vi "test_Add Array Format.vi"(8 "error in (no error)":errorcluster, 11 "TestCase in":refnum<class "Instrument Addon Scripting API Channels Unit Tests.lvclass">) -> (0 "error out":errorcluster, 3 "TestCase out":refnum<class "Instrument Addon Scripting API Channels Unit Tests.lvclass">)   [LabVIEW 2018, in "Instrument Addon Scripting API Channels Unit Tests.lvclass"]
uses:
  Instrument Addon Scripting API Channels Unit Tests.lvclass
  APIs/Scripting API/TypeDefs/Array Format Settings.ctl
  APIs/Scripting API/TypeDefs/Array Element.ctl
  Addon/Addon Shared/Types/Protocol Data Type.ctl
  Addon/Addon Shared/Types/Data Channel Type.ctl
  Instrument Addon Scripting API Channels Unit Tests.lvclass/Instrument Addon Scripting API Channels Unit Tests.ctl
  Addon/Addon Shared/SubVIs/Constants.vi
  <vilib>/NI/NI VeriStand Advanced SysDef API/_SubVIs/SysDef.Search.GUID.vi
  <vilib>/NI/NI VeriStand Advanced SysDef API/_SubVIs/SysDef.Search.GUIDs.vi
  APIs/Scripting API/Channels/Create Data Channel - Array - Format.vi
  <vilib>/NI Veristand/Custom Device API/Get Item Property (U16).vi
  <vilib>/NI Veristand/Custom Device API/Get Item Property (String).vi
  <vilib>/addons/_JKI Toolkits/VI Tester/TestCase.llb/TestCase.lvclass
  Instrument Addon Scripting API Test Assets/Instrument Addon Scripting API Test Assets.lvclass
  <vilib>/NI/NI VeriStand Advanced SysDef API/SysDef API/Advanced System Definition.lvlib
  Addon/Addon Shared/Instrument Addon Shared.lvlib
  APIs/Scripting API/Instrument Addon Scripting API.lvlib
  <vilib>/NI Veristand/Custom Device API/Custom Device API.lvlib
  C:/Program Files (x86)/National Instruments/LabVIEW 2018/vi.lib/addons/_JKI Toolkits/VI Tester/TestCase.llb/TestCase.lvclass
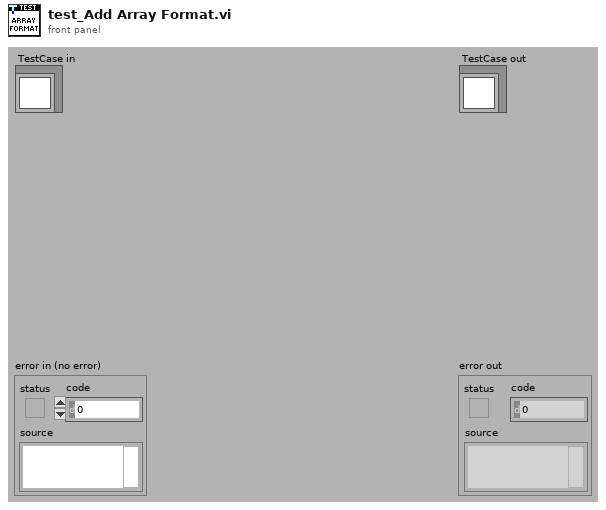
[diagram p1: front panel]
types:
  T1 = typedef "Instrument Addon Scripting API.lvlib/Array Format Settings.ctl" = cluster{"Elements":T2[], "Format String":string, "Delimiter":string}
  T2 = typedef "Instrument Addon Scripting API.lvlib/Array Element.ctl" = cluster{"Name":string, "Default Value":dbl, "Units":string}
  T3 = typedef "Instrument Addon Shared.lvlib/Data Channel Type.ctl" = enum16{"Format", "Comparison", "Type Cast", "Enumerated List"}
  T4 = typedef "Instrument Addon Shared.lvlib/Protocol Data Type.ctl" = enum16{"Single Channel", "Array"}
  T5 = typedef "Custom Device API.lvlib/Custom Device Item Ref.ctl" = u64
  T6 = typedef "Advanced System Definition.lvlib/TreeItem.Info.ctl" = cluster{"Name":string, "Description":string, "GUID":string, "Is Channel":bool, "Channel":T7, "Is Waveform":bool, "Waveform":T9}
  T7 = typedef "Custom Device API.lvlib/Custom Device Channel.ctl" = cluster{"Type":T8, "Units":string, "Default Value":dbl, "Faultable":bool, "Scalable":bool}
  T8 = typedef "Custom Device API.lvlib/Custom Device Channel Type.ctl" = enum16{"Input", "Output"}
  T9 = typedef "Custom Device API.lvlib/Custom Device Waveform.ctl" = cluster{"Data Type":T10, "Units":string}
  T10 = typedef "Custom Device API.lvlib/Custom Device Waveform DataType.ctl" = enum16{"Double", "Complex Double"}
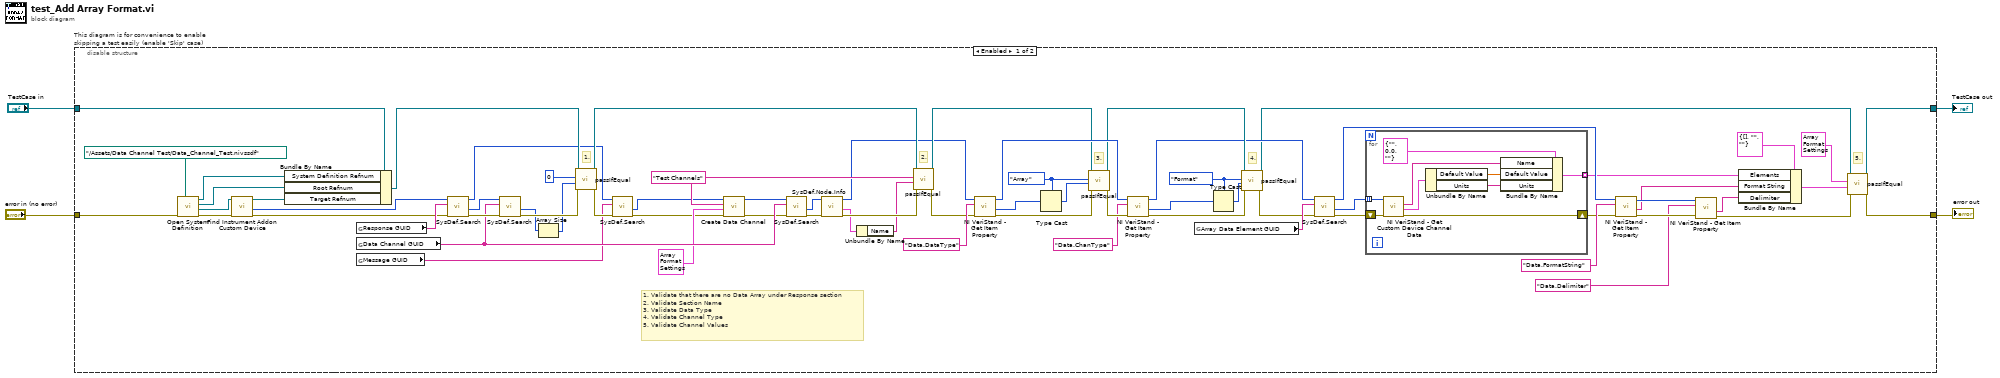
[diagram p0: block diagram]
diagram:
  n1 = disable-structure "This diagram is for convenience to enable skipping a test easily (enable 'Skip' case)" shown="Enabled" {
    disable-tunnel: "TestCase in" -> [w36 w88]
    disable-tunnel: [w49 w86] -> w1
    disable-tunnel: [w50 w87] -> w3
    disable-tunnel: "error in (no error)" -> [w72 w85]
    frame Enabled {
      w14 = Data_Channel_Type."Format" ("Channel Type")
      w19 = Protocol_Data_Type."Array" ("Data Type")
      w61 = "Test Channels" ("Name")
      # "1. Validate that there are no Data Array under Response section\n2. Validate Section Name\n3. Validate Data Type\n4. Validate Channel Type\n5. Validate Channel Values"
      # "4."
      # "3."
      # "5."
      # "2."
      # "1."
      n2 = call "Open System Definition.vi"("error in (no error)"=w72, "System Definition File"=path "../Assets/Data Channel Test/Data_Channel_Test.nivssdf") -> ("error out"=w75:errorcluster, "Target Refnum"=w74:refnum<k24>, "Root Refnum"=w34:refnum<k24>, "System Definition Refnum"=w35:refnum<k24>)  [unwired: 6 in]
      n3 = call "Find Instrument Addon Custom Device.vi"("error in"=w75, "target in"=w74) -> ("error out"=w32:errorcluster, "NodeID"=w71:u64, "target out"=w33:refnum<k24>)  [unwired: 7 in]
      n4 = Bundle By Name(cluster=w36, "System Definition Refnum"=w35, "Root Refnum"=w34, "Target Refnum"=w33) -> (w31:refnum<class "Instrument Addon Scripting API Channels Unit Tests.lvclass">)
      n5 = global read "Constants.vi" "Response GUID"() -> (w70:string)
      n6 = global read "Constants.vi" "Data Channel GUID"() -> (w67:string)
      n7 = global read "Constants.vi" "Message GUID"() -> (w28:string)
      n8 = call-poly <vilib>:"SysDef.Search.vi"("error in (no error)"=w32, "GUID"=w70, "nodeID"=w71) -> ("error out"=w68:errorcluster, "Value out"=w69:u64, "nodeID out"=w27:u64)  [unwired: 5 in, 1 out]
      n9 = call-poly <vilib>:"SysDef.Search.vi"("error in (no error)"=w68, "GUID"=w67, "nodeID"=w69) -> ("error out"=w65:errorcluster, "Values Out"=w64:u64[])  [unwired: 5 in, 2 out]
      n10 = Array Size(array=w64) -> (size(s)=w63:i32)
      n11 = call-dynamic "passIfEqual.vi"("error in (no error)"=w65, "y"=w63, "x"=0 ("size(s)"), "TestCase in"=w31) -> ("error out"=w30:errorcluster, "TestCase out"=w66:refnum<class "Instrument Addon Scripting API Channels Unit Tests.lvclass">)  [unwired: 6 in]
      n12 = call-poly <vilib>:"SysDef.Search.vi"("error in (no error)"=w30, "GUID"=w28, "nodeID"=w27) -> ("error out"=w29:errorcluster, "Value out"=w26:u64)  [unwired: 5 in, 2 out]
      n13 = call-poly "Create Data Channel.vi"("Error In"=w29, "Settings"=T1 {"Elements"=[{"Name"="Rate", "Default Value"=50.0, "Units"="Hz"}, {"Name"="Time", "Default Value"=25.0, "Units"="ms"}], "Format String"="%03", "Delimiter"=","}, "Name"=w61, "Message Refnum In"=w26) -> ("Error Out"=w60:errorcluster, "Message Refnum Out"=w59:T5)  [unwired: 5 in, 1 out]
      n14 = call-poly <vilib>:"SysDef.Search.vi"("error in (no error)"=w60, "GUID"=w67, "nodeID"=w59) -> ("error out"=w58:errorcluster, "Value out"=w57:u64)  [unwired: 5 in, 2 out]
      n15 = call <vilib>:"SysDef.Node.Info.vi"("error in (no error)"=w58, "nodeID"=w57) -> ("error out"=w56:errorcluster, "Item Info"=w55:T6, "nodeID out"=w8:u64)  [unwired: 6 in, 1 out]
      n16 = Unbundle By Name(w55) -> ("Name"=w54:string)
      n17 = call-dynamic "passIfEqual.vi"("error in (no error)"=w56, "y"=w54, "x"=w61, "TestCase in"=w66) -> ("error out"=w9:errorcluster, "TestCase out"=w11:refnum<class "Instrument Addon Scripting API Channels Unit Tests.lvclass">)  [unwired: 6 in]
      n18 = call-poly <vilib>:"NI VeriStand - Get Item Property.vi"("error in (no error)"=w9, "Property Name"="Data.DataType", "Item Ref in"=w8) -> ("error out"=w22:errorcluster, "Value"=w21:u16, "Item Ref out"=w13:T5)  [unwired: 5 in, 1 out]
      n19 = Type Cast(type=w19, x=w21) -> (*(type *) &x=w20:T4)
      n20 = call-dynamic "passIfEqual.vi"("error in (no error)"=w22, "y"=w20, "x"=w19, "TestCase in"=w11) -> ("error out"=w18:errorcluster, "TestCase out"=w10:refnum<class "Instrument Addon Scripting API Channels Unit Tests.lvclass">)  [unwired: 6 in]
      n21 = call-poly <vilib>:"NI VeriStand - Get Item Property.vi"("error in (no error)"=w18, "Property Name"="Data.ChanType", "Item Ref in"=w13) -> ("error out"=w17:errorcluster, "Value"=w16:u16, "Item Ref out"=w7:T5)  [unwired: 5 in, 1 out]
      n22 = global read "Constants.vi" "Array Data Element GUID"() -> (w52:string)
      n23 = Type Cast(type=w14, x=w16) -> (*(type *) &x=w15:T3)
      n24 = call-dynamic "passIfEqual.vi"("error in (no error)"=w17, "y"=w15, "x"=w14, "TestCase in"=w10) -> ("error out"=w6:errorcluster, "TestCase out"=w5:refnum<class "Instrument Addon Scripting API Channels Unit Tests.lvclass">)  [unwired: 6 in]
      n25 = call-poly <vilib>:"SysDef.Search.vi"("error in (no error)"=w6, "GUID"=w52, "nodeID"=w7) -> ("error out"=w53:errorcluster, "Values Out"=w51:u64[], "nodeID out"=w46:u64)  [unwired: 5 in, 1 out]
      n26 = for {
        shift-right: [w76] -> w47
        shift-left: w53 -> [w83]
        tunnel: w51 -> [w84] mode=indexing
        tunnel: [w77] -> w45 mode=indexing
        n27 = call <vilib>:"NI VeriStand - Get Custom Device Channel Data.vi"("error in (no error)"=w83, "Channel Ref in"=w84) -> ("error out"=w76:errorcluster, "Channel"=w80:T7, "Channel Name"=w81:string)  [unwired: 4 in, 3 out]
        n28 = Unbundle By Name(w80) -> ("Default Value"=w78:dbl, "Units"=w79:string)
        n29 = Bundle By Name(cluster=T2 {"Name"="", "Default Value"=0.0, "Units"=""} ("Array Element"), "Name"=w81, "Default Value"=w78, "Units"=w79) -> (w77:T2)
      }
      n30 = call-poly <vilib>:"NI VeriStand - Get Item Property.vi"("error in (no error)"=w47, "Property Name"="Data.FormatString", "Item Ref in"=w46) -> ("error out"=w44:errorcluster, "Value"=w38:string, "Item Ref out"=w43:T5)  [unwired: 5 in, 1 out]
      n31 = call-poly <vilib>:"NI VeriStand - Get Item Property.vi"("error in (no error)"=w44, "Property Name"="Data.Delimiter", "Item Ref in"=w43) -> ("error out"=w40:errorcluster, "Value"=w41:string)  [unwired: 5 in, 2 out]
      n32 = Bundle By Name(cluster=T1 {"Elements"=[], "Format String"="", "Delimiter"=""} ("Settings"), "Elements"=w45, "Format String"=w38, "Delimiter"=w41) -> (w25:T1)
      n33 = call-dynamic "passIfEqual.vi"("error in (no error)"=w40, "y"=w25, "x"=T1 {"Elements"=[{"Name"="Rate", "Default Value"=50.0, "Units"="Hz"}, {"Name"="Time", "Default Value"=25.0, "Units"="ms"}], "Format String"="%03", "Delimiter"=","} ("Settings"), "TestCase in"=w5) -> ("error out"=w50:errorcluster, "TestCase out"=w49:refnum<class "Instrument Addon Scripting API Channels Unit Tests.lvclass">)  [unwired: 6 in]
    }
    frame Disabled {
      # "skip test result while test is under development"
      n34 = call <vilib>:"skip.vi"("error in (no error)"=w85, "TestCase in"=w88) -> ("error out"=w87:errorcluster, "TestCase out"=w86:refnum<class "Instrument Addon Scripting API Channels Unit Tests.lvclass">)  [unwired: 8 in]
    }
  }
  "error out" <- w3
  "TestCase out" <- w1
